vi "Raster.vi"(10 "Pixel Data in":u32[][](array[numeric]), 11 "Scene in":refnum<class "Scene.lvclass">) -> (2 "Pixel Data out":u32[][](array[numeric]), 3 "Scene out":refnum<class "Scene.lvclass">)   [LabVIEW 2020, in "Scene.lvclass"]
uses:
  Scene.lvclass
  Scene.lvclass/Scene.ctl
  Graphics/Libraries/3D/3D.lvlib
  edb3f0c2-b950-4a44-8897-096d76b30880.vi
  76d78098-f527-454b-a08a-aac5a717328f.vi
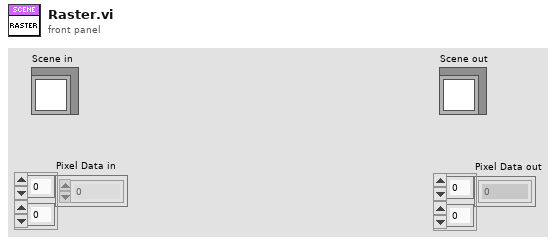
[diagram p1: front panel]
types:
  T1 = typedef "3D.lvlib/Triangle.ctl" = cluster{"Vertex 1":T2, "Vertex 2":T2, "Vertex 3":T2, "Alpha":dbl, "Alpha Blending Enabled":bool, "Colour":u32, "Material":T5}
  T2 = typedef "3D.lvlib/Vertex.ctl" = cluster{"Position":T3, "UV":T4, "Colour":u32}
  T3 = typedef "3D.lvlib/Vector 3D.ctl" = cluster{"x":sgl, "y":sgl, "z":sgl}
  T4 = typedef "Raster.lvlib/UV.ctl" = cluster{"u":sgl, "v":sgl}
  T5 = typedef "3D.lvlib/Material.ctl" = cluster{"Diffuse Colour":u32, "Texture":T6}
  T6 = typedef "Raster.lvlib/Texture.ctl" = cluster{"Pixels":refnum<data-value>, "Size":T7}
  T7 = typedef "Raster.lvlib/Rectangle Dimensions.ctl" = cluster{"Width":u32, "Height":u32}
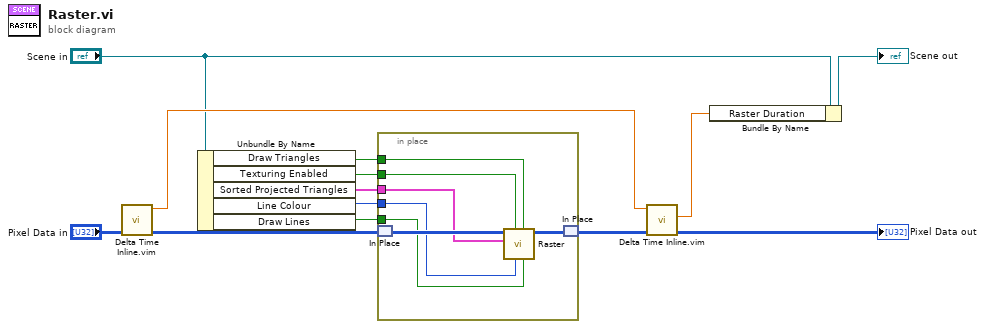
[diagram p0: block diagram]
diagram:
  n1 = call "Delta Time Inline.vim"("value in"="Pixel Data in") -> ("value out"=w9:u32[][], "Relative Seconds out [s]"=w13:dbl)  [unwired: 8 in, 1 out]
  n2 = Unbundle By Name("Scene in") -> ("Draw Triangles"=w4:bool, "Texturing Enabled"=w1:bool, "Sorted Projected Triangles"=w8:T1[], "Line Colour"=w3:u32, "Draw Lines"=w2:bool)
  n3 = in-place {
    in-place-border: w8 -> [w18]
    in-place-border: w4 -> [w17]
    in-place-border: w3 -> [w16]
    in-place-border: w2 -> [w15]
    in-place-border: w1 -> [w14]
    n4 = in-place-match #1(w9) -> (w20:u32[][])
    n5 = call "Raster.vi"("Draw Lines"=w15, "Draw Triangles"=w17, "Line Colour"=w16, "Textured"=w14, "Triangles Sorted"=w18, "Pixel Data in"=w20) -> ("Pixel Data out"=w19:u32[][])  [unwired: 5 in]
    n6 = in-place-match #1(w19) -> (w12:u32[][])
  }
  n7 = call "Delta Time Inline.vim"("value in"=w12, "Relative Seconds in [s]"=w13) -> ("value out"=→"Pixel Data out":u32[][], "Delta Time [s]"=w5:dbl)  [unwired: 7 in, 1 out]
  n8 = Bundle By Name(cluster="Scene in", "Raster Duration"=w5) -> (→"Scene out":refnum<class "Scene.lvclass">)
